vi "GoBang_RemoveStonesFromSubArray.vi"(1 "4x4 array in":u8[][](array[numeric])=[[0, 0, 0, 0], [0, 0, 0, 0], [0, 0, 0, 0], [0, 0, 0, 0]]) -> (0 "4x4 array out":u8[][](array[numeric]))   [LabVIEW 2013, in "GoBang.lvlib"]
uses:
  GoBang.lvlib
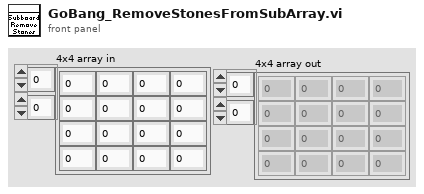
[diagram p1: front panel]
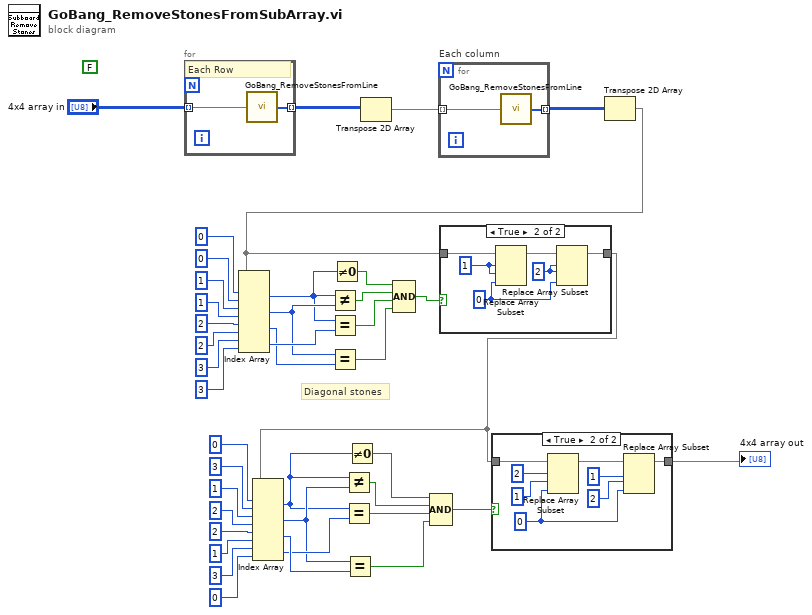
[diagram p0: block diagram]
diagram:
  (unwired) FALSE
  # "Diagonal stones"
  n1 = for {
    tunnel: "4x4 array in" -> [w43] mode=indexing
    tunnel: [w42] -> w32 mode=indexing
    # "Each Row"
    n2 = call "GoBang_RemoveStonesFromLine.vi"("line with 4 elements in"=w43) -> ("line with 4 elements out"=w42:u8[])
  }
  n3 = Transpose 2D Array(2D array=w32) -> (transposed array=w31:u8[][])
  n4 = for "Each column" {
    tunnel: w31 -> [w45] mode=indexing
    tunnel: [w44] -> w30 mode=indexing
    n5 = call "GoBang_RemoveStonesFromLine.vi"("line with 4 elements in"=w45) -> ("line with 4 elements out"=w44:u8[])
  }
  n6 = Transpose 2D Array(2D array=w30) -> (transposed array=w24:u8[][])
  n7 = Index Array(array=w24, index (row) #1=0 ("index (row)"), index (col) #1=0 ("disabled index (col)"), index (row) #2=1 ("index (row)"), index (col) #2=1 ("disabled index (col)"), index (row) #3=2 ("index (row)"), index (col) #3=2 ("disabled index (col)"), index (row) #4=3 ("index (row)"), index (col) #4=3 ("disabled index (col)")) -> (element #1=w4:u8, element #2=w8:u8, element #3=w28:u8, element #4=w29:u8)
  n8 = Not Equal?(x=w4, y=w8) -> (x != y?=w7:bool)
  n9 = Equal?(x=w4, y=w29) -> (x = y?=w27:bool)
  n10 = Equal?(x=w8, y=w28) -> (x = y?=w26:bool)
  n11 = Not Equal To 0?(x=w4) -> (x != 0?=w3:bool)
  n12 = Compound Arithmetic op=AND(w3, w7, w27, w26) -> (w25:bool)
  n13 = case shown="True" w25 {
    tunnel: w24 -> [w46 w52]
    tunnel: [w46 w47] -> w10
    frame False {
    }
    frame True {
      w49 = 2 ("index (row)")
      w48 = u8 0 ("new element/subarray")
      w51 = 1 ("index (row)")
      n14 = Replace Array Subset(array=w52, new element=w48, index (row)=w51, index (col)=w51) -> (w50:u8[][])
      n15 = Replace Array Subset(array=w50, new element=w48, index (row)=w49, index (col)=w49) -> (w47:u8[][])
    }
  }
  n16 = Index Array(array=w10, index (row) #1=0 ("index (row)"), index (col) #1=3 ("disabled index (col)"), index (row) #2=1 ("index (row)"), index (col) #2=2 ("disabled index (col)"), index (row) #3=2 ("index (row)"), index (col) #3=1 ("disabled index (col)"), index (row) #4=3 ("index (row)"), index (col) #4=0 ("disabled index (col)")) -> (element #1=w2:u8, element #2=w6:u8, element #3=w20:u8, element #4=w19:u8)
  n17 = Not Equal?(x=w2, y=w6) -> (x != y?=w5:bool)
  n18 = Equal?(x=w2, y=w19) -> (x = y?=w21:bool)
  n19 = Equal?(x=w6, y=w20) -> (x = y?=w22:bool)
  n20 = Not Equal To 0?(x=w2) -> (x != 0?=w1:bool)
  n21 = Compound Arithmetic op=AND(w1, w5, w21, w22) -> (w23:bool)
  n22 = case shown="True" w23 {
    tunnel: w10 -> [w53 w61]
    tunnel: [w53 w56] -> w9
    frame False {
    }
    frame True {
      w57 = u8 0 ("new element/subarray")
      n23 = Replace Array Subset(array=w61, new element=w57, index (row)=2, index (col)=1 ("disabled index (col)")) -> (w59:u8[][])
      n24 = Replace Array Subset(array=w59, new element=w57, index (row)=1 ("disabled index (row)"), index (col)=2 ("index (row)")) -> (w56:u8[][])
    }
  }
  "4x4 array out" <- w9
